vi "DispatchInterface_Get Tags_deleteme.vi"(8 "error in (no error)":errorcluster, 11 "DispatchInterface in":refnum<class "Interface_Dispatch.lvclass">) -> (0 "error out":errorcluster, 3 "DispatchInterface out":refnum<class "Interface_Dispatch.lvclass">)   [LabVIEW 2015]
uses:
  Interface_Dispatch.lvclass
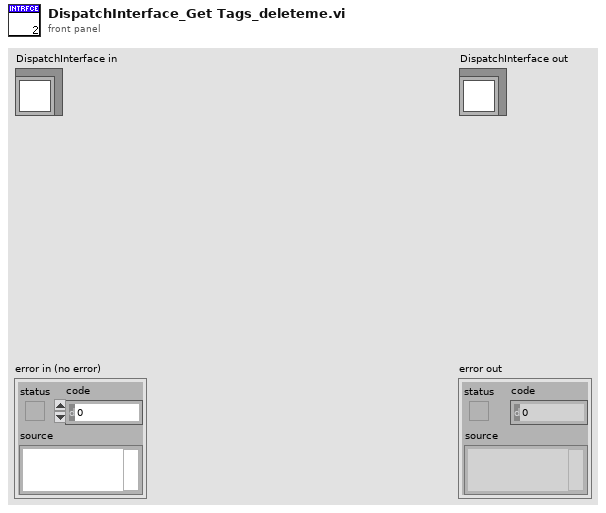
[diagram p1: front panel]
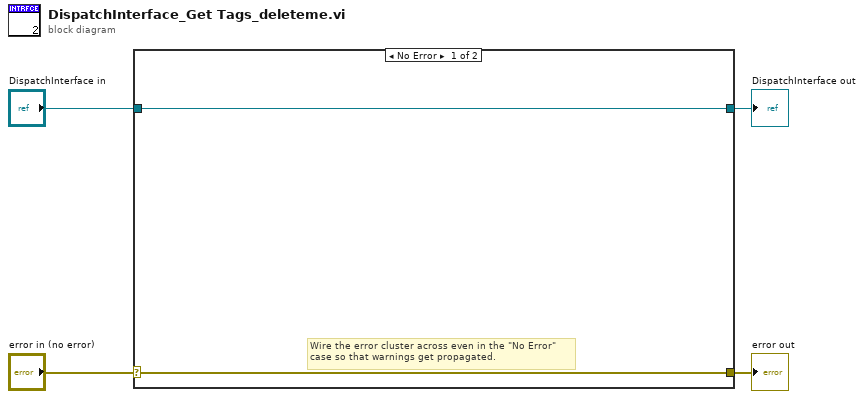
[diagram p0: block diagram]
diagram:
  n1 = case shown="No Error" "error in (no error)" {
    selector: "error in (no error)" -> [w5 w8]
    tunnel: [w5 w8] -> w3
    tunnel: [w6 w7] -> w1
    tunnel: "DispatchInterface in" -> [w6 w7]
    frame No Error {
      # "Wire the error cluster across even in the \"No Error\"\ncase so that warnings get propagated."
    }
    frame Error {
    }
  }
  "error out" <- w3
  "DispatchInterface out" <- w1
